vi "OSAread.vi"() -> (0 "power":dbl[](array[numeric]), 1 "length":dbl[](array[numeric]))   [LabVIEW 2019]
panel:
  out "array":dbl[](array[numeric])
  out "output array":dbl[][](array[numeric])
  out "Characters Read 2":string
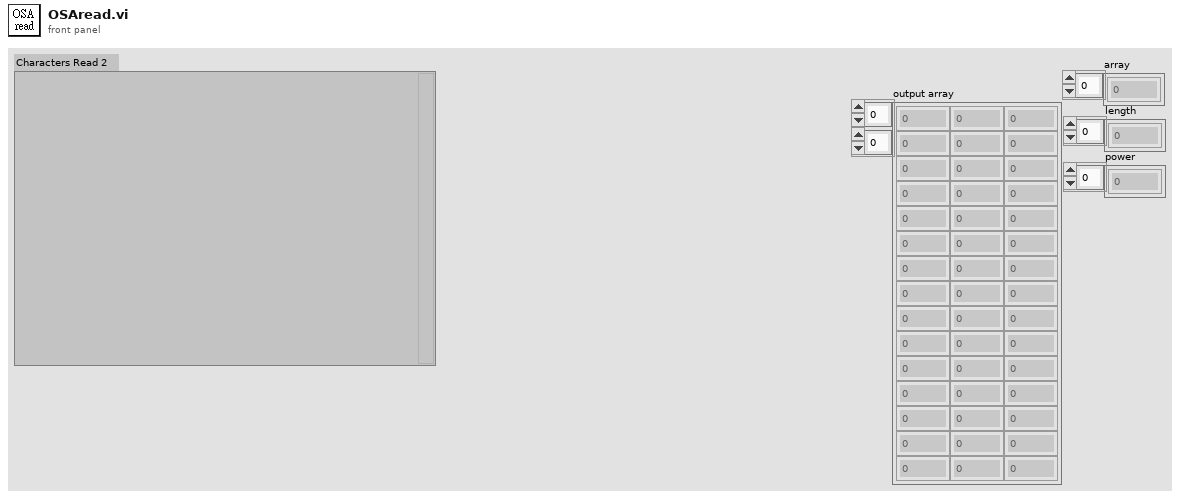
[diagram p1: front panel]
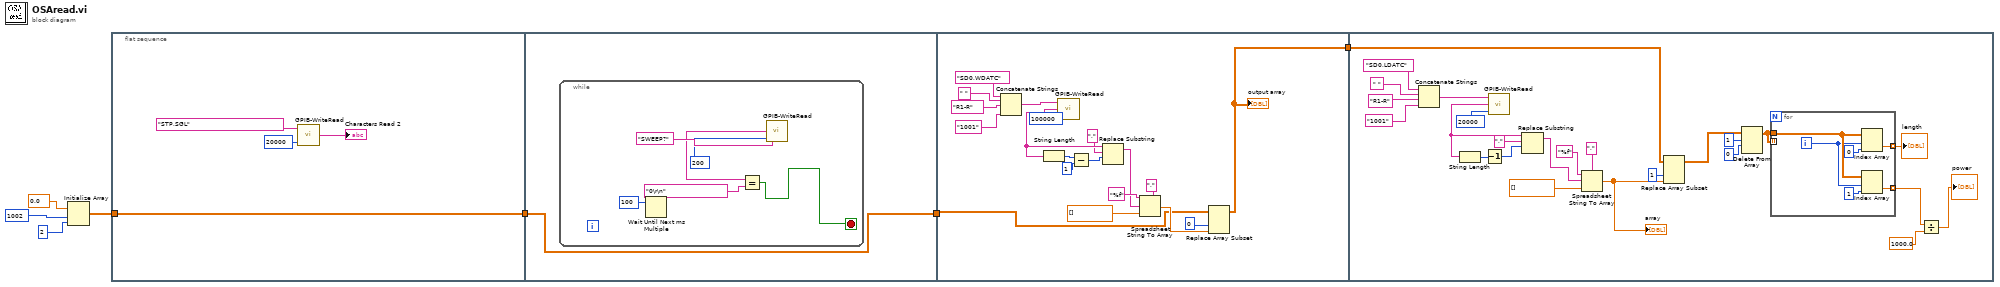
[diagram p0: block diagram]
diagram:
  n1 = Initialize Array(0.0 ("element"), 1002 ("dimension size"), 2 ("dimension size")) -> (w4:dbl[][])
  n2 = flat-sequence {
    tunnel: w4 -> [w10]
    tunnel: [w10] -> w3
    tunnel: w3 -> [w12]
    tunnel: [w12] -> w2
    tunnel: w2 -> [w21]
    tunnel: [w19] -> w1
    tunnel: w1 -> [w46]
    frame #0 {
      n3 = call "GPIB-WriteRead.vi"("# bytes\nto read"=20000 ("# bytes\nto read"), "Characters to Write"="STP,SGL") -> ("Characters Read"=→"Characters Read 2":string)  [unwired: 2 out]
    }
    frame #1 {
      n4 = while {
        stop <- w18 stop-if-true
        n5 = Wait Until Next ms Multiple(millisecond multiple=100) -> ()  [unwired: 1 out]
        n6 = call "GPIB-WriteRead.vi"("# bytes\nto read"=200 ("# bytes\nto read"), "Characters to Write"="SWEEP?") -> ("Characters Read"=w15:string)  [unwired: 2 out]
        n7 = Equal?(x=w15, y="0\r\n" ("Characters Read")) -> (x = y?=w18:bool)
      }
    }
    frame #2 {
      n8 = Concatenate Strings("SD0,WDATC", " ", "R1-R", "1001") -> (w32:string)
      n9 = call "GPIB-WriteRead.vi"("# bytes\nto read"=100000, "Characters to Write"=w32) -> ("Characters Read"=w27:string)  [unwired: 2 out]
      n10 = String Length(string=w27) -> (length=w25:i32)
      n11 = Subtract(x=w25, y=1) -> (x-y=w23:i32)
      n12 = Replace Substring(3:w23, 4:",", 5:w27) -> (1:w22:string)  [unwired: 2 out]
      n13 = Spreadsheet String To Array(delimiter (Tab)=",", format string="%f", spreadsheet string=w22, array type (2D Dbl)=dbl[] []) -> (array=w30:dbl[])
      n14 = Replace Array Subset(array=w21, new element=w30, index (col)=0 ("disabled index (col)")) -> (w19:dbl[][])  [unwired: 1 in]
      "output array" <- w19
    }
    frame #3 {
      n15 = Concatenate Strings("SD0,LDATC", " ", "R1-R", "1001") -> (w59:string)
      n16 = call "GPIB-WriteRead.vi"("# bytes\nto read"=20000 ("# bytes\nto read"), "Characters to Write"=w59) -> ("Characters Read"=w51:string)  [unwired: 2 out]
      n17 = String Length(string=w51) -> (length=w52:i32)
      n18 = Decrement(x=w52) -> (x-1=w49:i32)
      n19 = Replace Substring(3:w49, 4:",", 5:w51) -> (1:w48:string)  [unwired: 2 out]
      n20 = Spreadsheet String To Array(delimiter (Tab)=",", format string="%f", spreadsheet string=w48, array type (2D Dbl)=dbl[] []) -> (array=w55:dbl[])
      "array" <- w55
      n21 = Replace Array Subset(array=w46, new element=w55, index (col)=1) -> (w42:dbl[][])  [unwired: 1 in]
      n22 = Delete From Array(array=w42, length=1, index (row)=0) -> (array with subset deleted=w43:dbl[][])  [unwired: 1 in, 1 out]
      n23 = for {
        tunnel: w43 -> [w68]
        tunnel: w43 -> [_] mode=indexing
        tunnel: [w64] -> w41 mode=indexing
        tunnel: [w63] -> w39 mode=indexing
        i -> [w66]
        n24 = Index Array(array=w68, index (row)=w66, index (col)=0 ("disabled index (row)")) -> (element=w64:dbl)
        n25 = Index Array(array=w68, index (row)=w66, index (col)=1 ("disabled index (row)")) -> (element=w63:dbl)
      }
      "length" <- w41
      n26 = Divide(x=w39, y=1000.0) -> (x/y=→"power":dbl[])
    }
  }
